vi "act-0010-3-cor.vi"() -> ()   [LabVIEW 2010]
uses:
  lv_01/lv_01.lvlib
panel:
  in  "Choix (K ou F ou C)":string
  out "affichage":dbl caption="Temp simulée en°K"
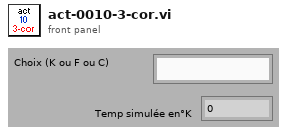
[diagram p1: front panel]
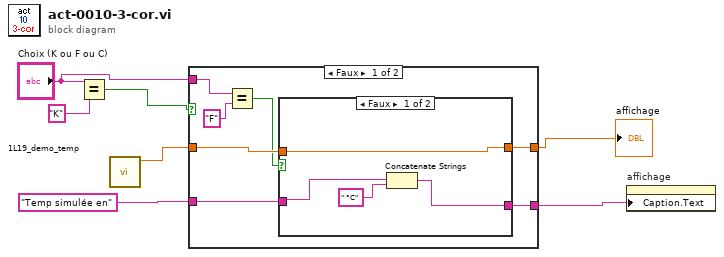
[diagram p0: block diagram]
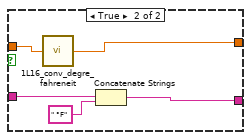
[diagram p2: hidden frame]
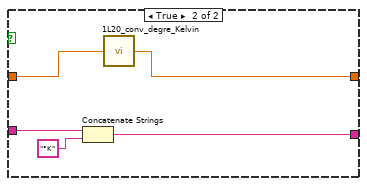
[diagram p3: hidden frame]
diagram:
  n1 = Equal?(x="Choix (K ou F ou C)", y="K") -> (x = y?=w2:bool)
  n2 = call "1L19_demo_temp.vi"() -> ("temp"=w7:dbl)  [unwired: 6 in, 1 out]
  n3 = case shown="Faux" w2 {
    tunnel: w7 -> [w14 w25]
    tunnel: "Temp simulée en" -> [w13 w27]
    tunnel: [w12 w26] -> w4
    tunnel: [w11 w24] -> w5
    tunnel: "Choix (K ou F ou C)" -> [w10 _]
    frame False {
      n4 = Equal?(x=w10, y="F") -> (x = y?=w8:bool)
      n5 = case shown="Faux" w8 {
        tunnel: w14 -> [w18 w23]
        tunnel: w13 -> [w16 w22]
        tunnel: [w15 w20] -> w12
        tunnel: [w18 w19] -> w11
        frame False {
          n6 = Concatenate Strings(w16, " °C" ("Étiquette.Texte")) -> (w15:string)
        }
        frame True {
          n7 = call "1L16_conv_degre_fahreneit.vi"("Deg C"=w23) -> ("Deg F"=w19:dbl)
          n8 = Concatenate Strings(w22, " °F" ("Étiquette.Texte")) -> (w20:string)
        }
      }
    }
    frame True {
      n9 = Concatenate Strings(w27, "°K" ("Étiquette.Texte")) -> (w26:string)
      n10 = call "1L20_conv_degre_Kelvin.vi"("Deg C"=w25) -> ("Deg K"=w24:dbl)
    }
  }
  "affichage" <- w5
  n11 = property on="affichage" class="NumDig (strict)"("Caption.Text"=w4) -> ()  [unwired: 2 in, 2 out]
